vi "DuplicatesInStringArray_.vi"(10 "String array":string[](array[string])) -> (2 "duplicates?":bool)   [LabVIEW 2013]
doc: "Check a string array for duplicate entries."
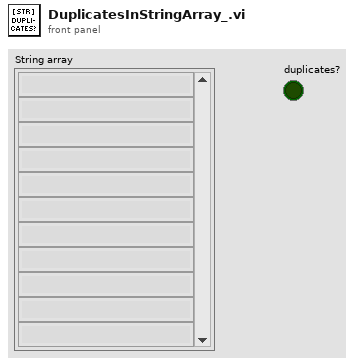
[diagram p1: front panel]
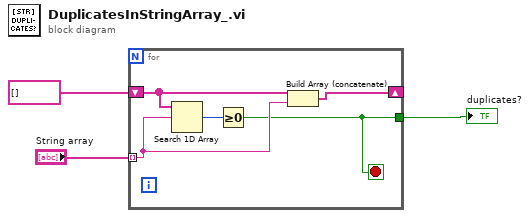
[diagram p0: block diagram]
diagram:
  n1 = for {
    tunnel: "String array" -> [w6] mode=indexing
    shift-right: [w5] -> _
    shift-left: string[] [] ("String array") -> [w7]
    tunnel: [w4] -> w1
    stop <- w4 stop-if-true
    n2 = Search 1D Array(1D array=w7, element=w6) -> (index of element=w8:i32)  [unwired: 1 in]
    n3 = Greater Or Equal To 0?(x=w8) -> (x >= 0?=w4:bool)
    n4 = Build Array (concatenate)(w7, w6) -> (w5:string[])
  }
  "duplicates?" <- w1
